vi "Check Amount of Pyramid Levels.vi"(6 "Image Type":T1=2 items=["Grayscale (U8)", "Grayscale (I16)", "Grayscale (SGL)", "Complex (CSG)", "RGB (U32)", "HSL (U32)", "RGB (U64)", "Grayscale (U16)"], 8 "error in (no error)":errorcluster, 11 "Refnum in":T2) -> (0 "error out":errorcluster, 2 "Image Dup":T2, 3 "Pyr Levels":i32)   [LabVIEW 2023]
uses:
  <vilib>/vision/Image Controls.llb/IMAQ Image.ctl
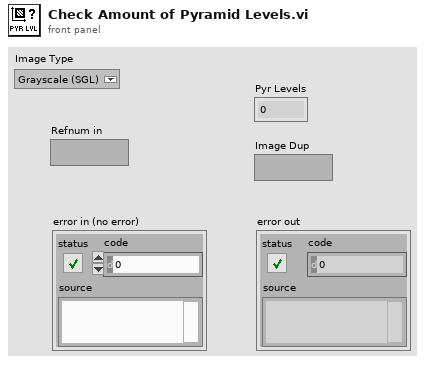
[diagram p1: front panel]
types:
  T1 = typedef "Image Type" = u32
  T2 = typedef "IMAQ Image.ctl" = refnum<image>
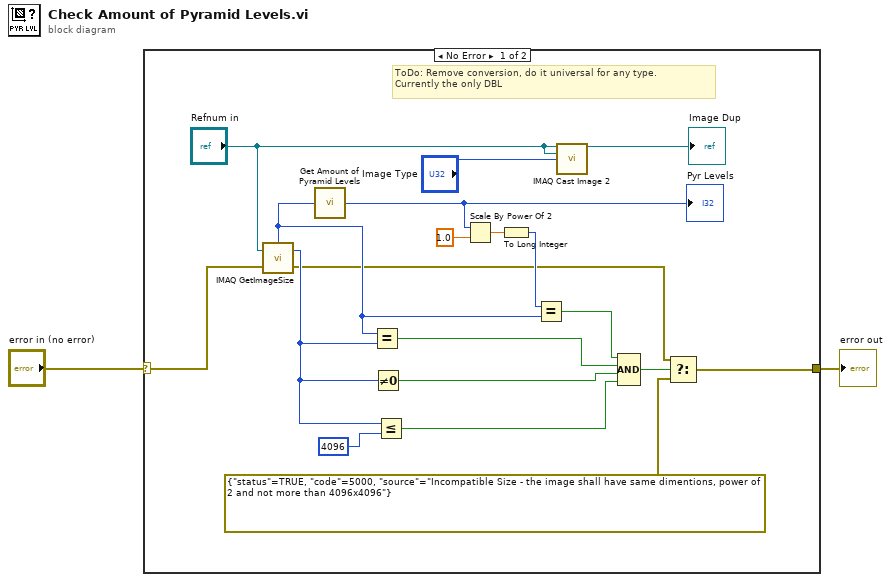
[diagram p0: block diagram]
diagram:
  n1 = case shown="No Error" "error in (no error)" {
    selector: "error in (no error)" -> [w3 w22]
    tunnel: [w8 w22] -> w2
    frame No Error {
      # "ToDo: Remove conversion, do it universal for any type.\nCurrently the only DBL"
      n2 = call "IMAQ GetImageSize"("Image"="Refnum in", "error in (no error)"=w3) -> ("Y Resolution"=w18:i32, "X Resolution"=w15:i32, "error out"=w9:errorcluster)  [unwired: 2 in]
      n3 = call "Get Amount of Pyramid Levels.vi"("X Resolution"=w15) -> ("Pyr Levels"=w20:i32)
      "Pyr Levels" <- w20
      n4 = Equal?(x=w15, y=w18) -> (x = y?=w13:bool)
      n5 = Not Equal To 0?(x=w18) -> (x != 0?=w12:bool)
      n6 = Less Or Equal?(x=w18, y=4096) -> (x <= y?=w11:bool)
      n7 = Scale By Power Of 2(n=w20, x=1.0) -> (x*2^n=w19:dbl)
      n8 = To Long Integer(number=w19) -> (32bit integer=w16:i32)
      n9 = Equal?(x=w16, y=w15) -> (x = y?=w14:bool)
      n10 = call "IMAQ Cast Image 2"("Image Src"="Refnum in", "Image Dst"="Refnum in", "Image Type"="Image Type") -> ("Image Dst Out"=→"Image Dup":T2)  [unwired: 11 in, 1 out]
      n11 = Compound Arithmetic op=AND(w14, w13, w12, w11) -> (w10:bool)
      n12 = Select(t=w9, s=w10, f=errorcluster {"status"=TRUE, "code"=5000, "source"="Incompatible Size - the image shall have same dimentions, power of 2 and not more than 4096x4096"}) -> (s? t:f=w8:errorcluster)
    }
    frame Error {
    }
  }
  "error out" <- w2
